vi "TabControl.vi"(0 "Ref In":refnum<vi>[](array[refnum]), 5 "SP Ref array in":refnum<vi>[](array[refnum]), 7 "Ctl Refnum":refnum<vi>, 11 "error in (no error)":errorcluster) -> (4 "Ref Out":refnum<vi>[](array[refnum]), 6 "SP Ref array out":refnum<vi>[](array[refnum]), 8 "InsertedVI":refnum<vi>, 10 "SubPnl Refnum":refnum<vi>, 15 "error out":errorcluster)   [LabVIEW 2016, in "Drona basic.lvlib"]
doc: "This VI gets the all the control's references present in a tab"
uses:
  Drona basic.lvlib
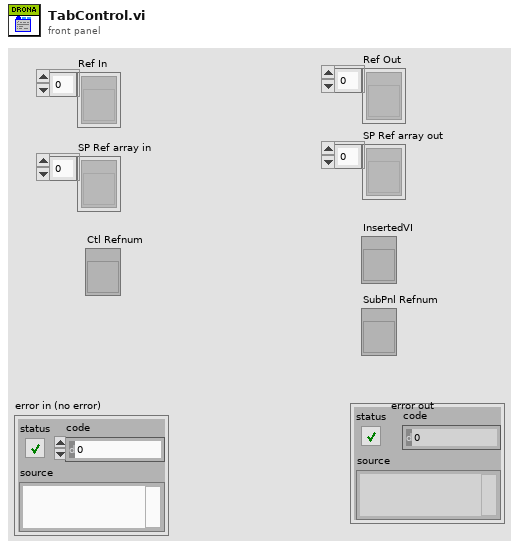
[diagram p1: front panel]
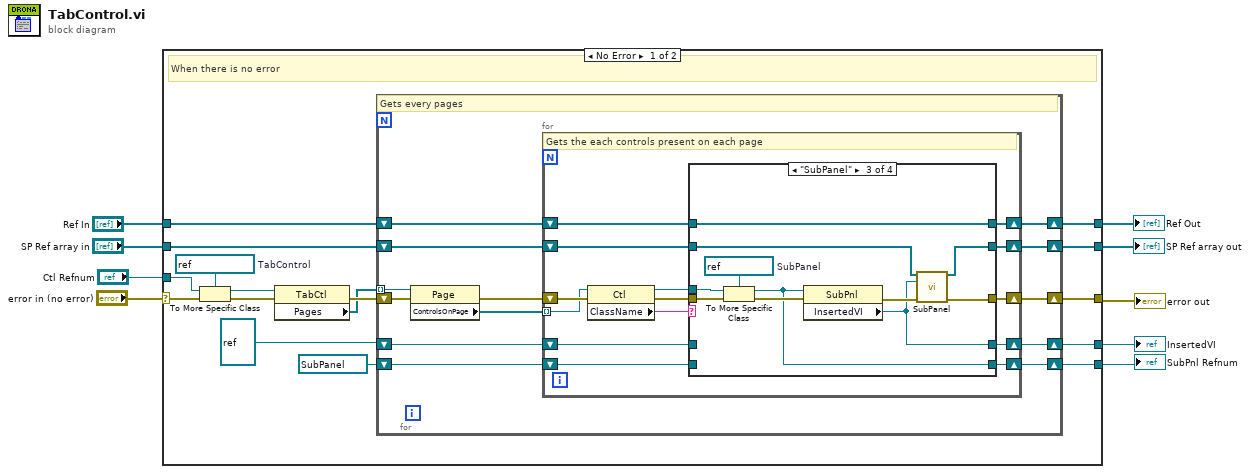
[diagram p0: block diagram]
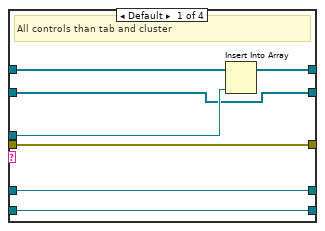
[diagram p2: hidden frame]
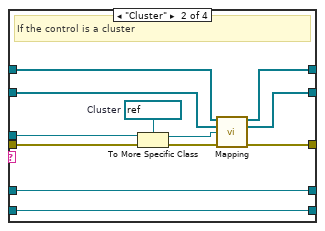
[diagram p3: hidden frame]
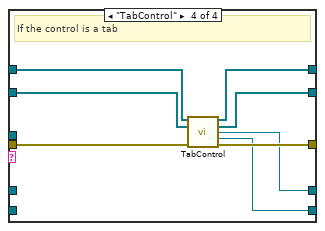
[diagram p4: hidden frame]
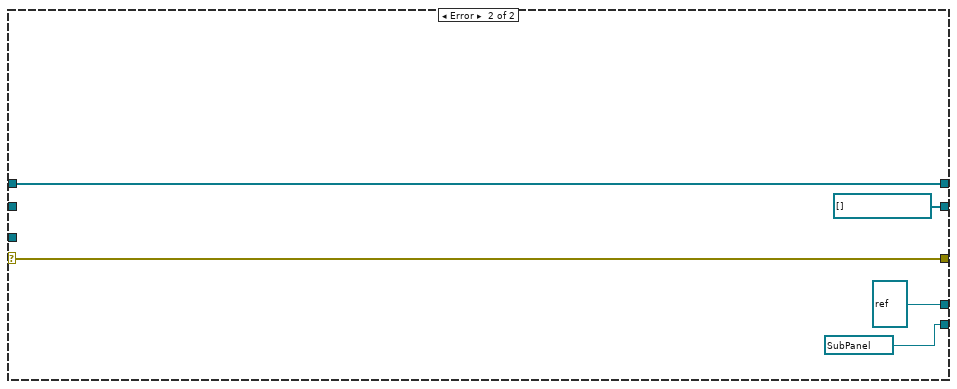
[diagram p5: hidden frame]
diagram:
  n1 = case shown="No Error" "error in (no error)" {
    selector: "error in (no error)" -> [w25 w95]
    tunnel: [w20 w95] -> w8
    tunnel: "Ctl Refnum" -> [w16 _]
    tunnel: "Ref In" -> [w17 w94]
    tunnel: [w18 w94] -> w5
    tunnel: "SP Ref array in" -> [w15 _]
    tunnel: [w14 refnum<vi>[] [] ("SP Ref array out")] -> w3
    tunnel: [w13 refnum<vi> refnum ("SubPnl Refnum")] -> w2
    tunnel: [w12 refnum<vi> refnum ("InsertedVI")] -> w1
    frame No Error {
      w21 = refnum<vi> refnum  # TabControl
      # "When there is no error"
      n2 = To More Specific Class(target class=w21, reference=w16, error in=w25) -> (specific class reference=w22:refnum<vi>, error out=w23:errorcluster)
      n3 = property class="TabCtl"(reference=w22, error in=w23) -> (error out=w24:errorcluster, "Pages"=w19:refnum<vi>[])  [unwired: 1 out]
      n4 = for {
        shift-right: [w37] -> w20
        shift-left: w24 -> [w38]
        tunnel: w19 -> [w34] mode=indexing
        shift-right: [w36] -> w18
        shift-left: w17 -> [w33]
        shift-right: [w30] -> w14
        shift-left: w15 -> [w31]
        shift-right: [w29] -> w13
        shift-left: refnum<vi> refnum ("SubPnl Refnum") -> [w26]
        shift-right: [w28] -> w12
        shift-left: refnum<vi> refnum ("InsertedVI") -> [w27]
        # "Gets every pages"
        n5 = property class="Page"(reference=w34, error in=w38) -> (error out=w35:errorcluster, "ControlsOnPage"=w32:refnum<vi>[])  [unwired: 1 out]
        n6 = for {
          shift-right: [w51] -> w37
          shift-left: w35 -> [w52]
          shift-right: [w49] -> w36
          shift-left: w33 -> [w50]
          tunnel: w32 -> [w45] mode=indexing
          shift-right: [w43] -> w30
          shift-left: w31 -> [w44]
          shift-right: [w42] -> w29
          shift-left: w26 -> [w39]
          shift-right: [w41] -> w28
          shift-left: w27 -> [w40]
          # "Gets the each controls present on each page"
          n7 = property class="Ctl"(reference=w45, error in=w52) -> (reference out=w47:refnum<vi>, error out=w46:errorcluster, "ClassName"=w48:string)
          n8 = case shown="\"SubPanel\"" w48 {
            tunnel: [w56 w71 w76 w89] -> w51
            tunnel: w50 -> [w59 w70 w72 w90]
            tunnel: w47 -> [w57 w69 w78 _]
            tunnel: [w58 w66 w72 w87] -> w49
            tunnel: w46 -> [w56 w65 w79 w88]
            tunnel: w44 -> [w53 w63 w74 w86]
            tunnel: [w53 w62 w73 w85] -> w43
            tunnel: [w54 w60 w77 w84] -> w42
            tunnel: [w55 w61 w75 w83] -> w41
            tunnel: w40 -> [w55 w61 _ _]
            tunnel: w39 -> [w54 w60 _ _]
            frame Default {
              # "All controls than tab and cluster"
              n9 = Insert Into Array(array=w59, new element=w57) -> (w58:refnum<vi>[])  [unwired: 1 in]
            }
            frame "Cluster" {
              w67 = refnum<vi> refnum  # Cluster
              # "If the control is a cluster"
              n10 = To More Specific Class(target class=w67, reference=w69, error in=w65) -> (specific class reference=w64:refnum<vi>, error out=w68:errorcluster)
              n11 = call "Mapping.vi"("Ref In"=w70, "SP Ref array in"=w63, "Clust Refnum"=w64, "error in (no error)"=w68) -> ("Ref Out"=w66:refnum<vi>[], "SP Ref array out"=w62:refnum<vi>[], "error out"=w71:errorcluster)  [unwired: 7 in, 2 out]
            }
            frame "SubPanel" {
              w81 = refnum<vi> refnum  # SubPanel
              n12 = To More Specific Class(target class=w81, reference=w78, error in=w79) -> (specific class reference=w77:refnum<vi>, error out=w82:errorcluster)
              n13 = property class="SubPnl"(reference=w77, error in=w82) -> (error out=w80:errorcluster, "InsertedVI"=w75:refnum<vi>)  [unwired: 1 out]
              n14 = call "SubPanel.vi"("Ref In"=w74, "VI reference"=w75, "error in (no error)"=w80) -> ("Ref Out"=w73:refnum<vi>[], "error out"=w76:errorcluster)  [unwired: 11 in]
            }
            frame "TabControl" {
              # "If the control is a tab"
              n15 = call "TabControl.vi"("Ref In"=w90, "SP Ref array in"=w86, "error in (no error)"=w88) -> ("Ref Out"=w87:refnum<vi>[], "SP Ref array out"=w85:refnum<vi>[], "InsertedVI"=w83:refnum<vi>, "SubPnl Refnum"=w84:refnum<vi>, "error out"=w89:errorcluster)  [unwired: 8 in]
            }
          }
        }
      }
    }
    frame Error {
    }
  }
  "error out" <- w8
  "Ref Out" <- w5
  "SP Ref array out" <- w3
  "SubPnl Refnum" <- w2
  "InsertedVI" <- w1
